vi "Bullet Markdown.vi"(8 "error in":errorcluster, 11 "File Path":path) -> (0 "error out":errorcluster, 2 "Wiki entry":string, 3 "Rendered metadata":string)   [LabVIEW 2020]
panel:
  out "result string":string
  out "String":string
  out "first subarray":string[](array[string])
  out "group/channel names":string[][](array[string])
  out "property values":variant[](array[variant])
  out "property names":string[](array[string])
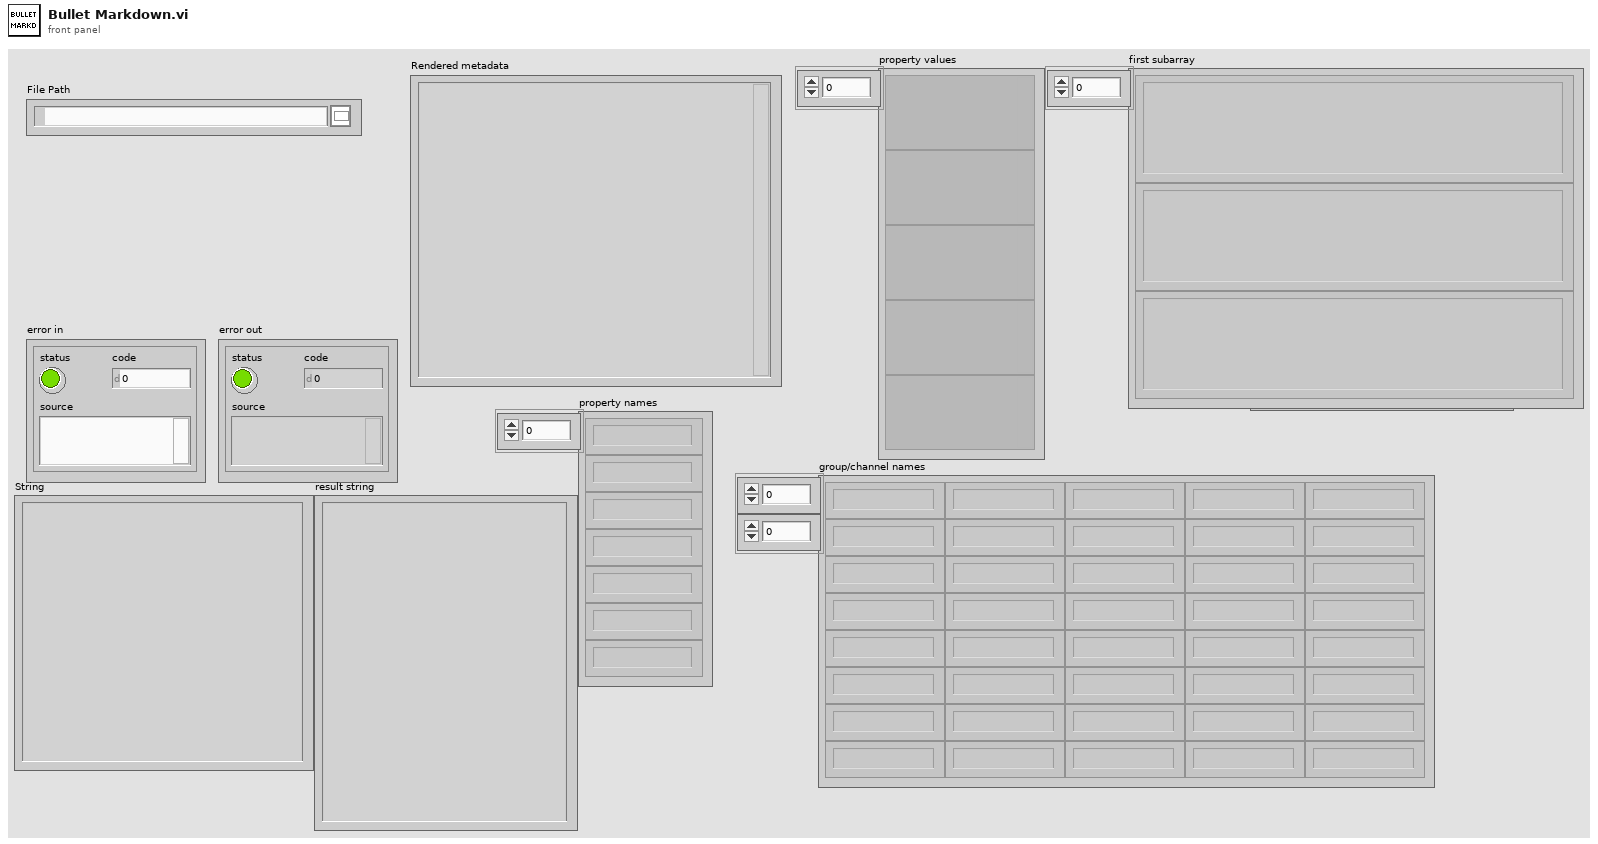
[diagram p1: front panel]
types:
  T1 = enum16{"open", "open or create", "create or replace", "create", "open (read-only)"}
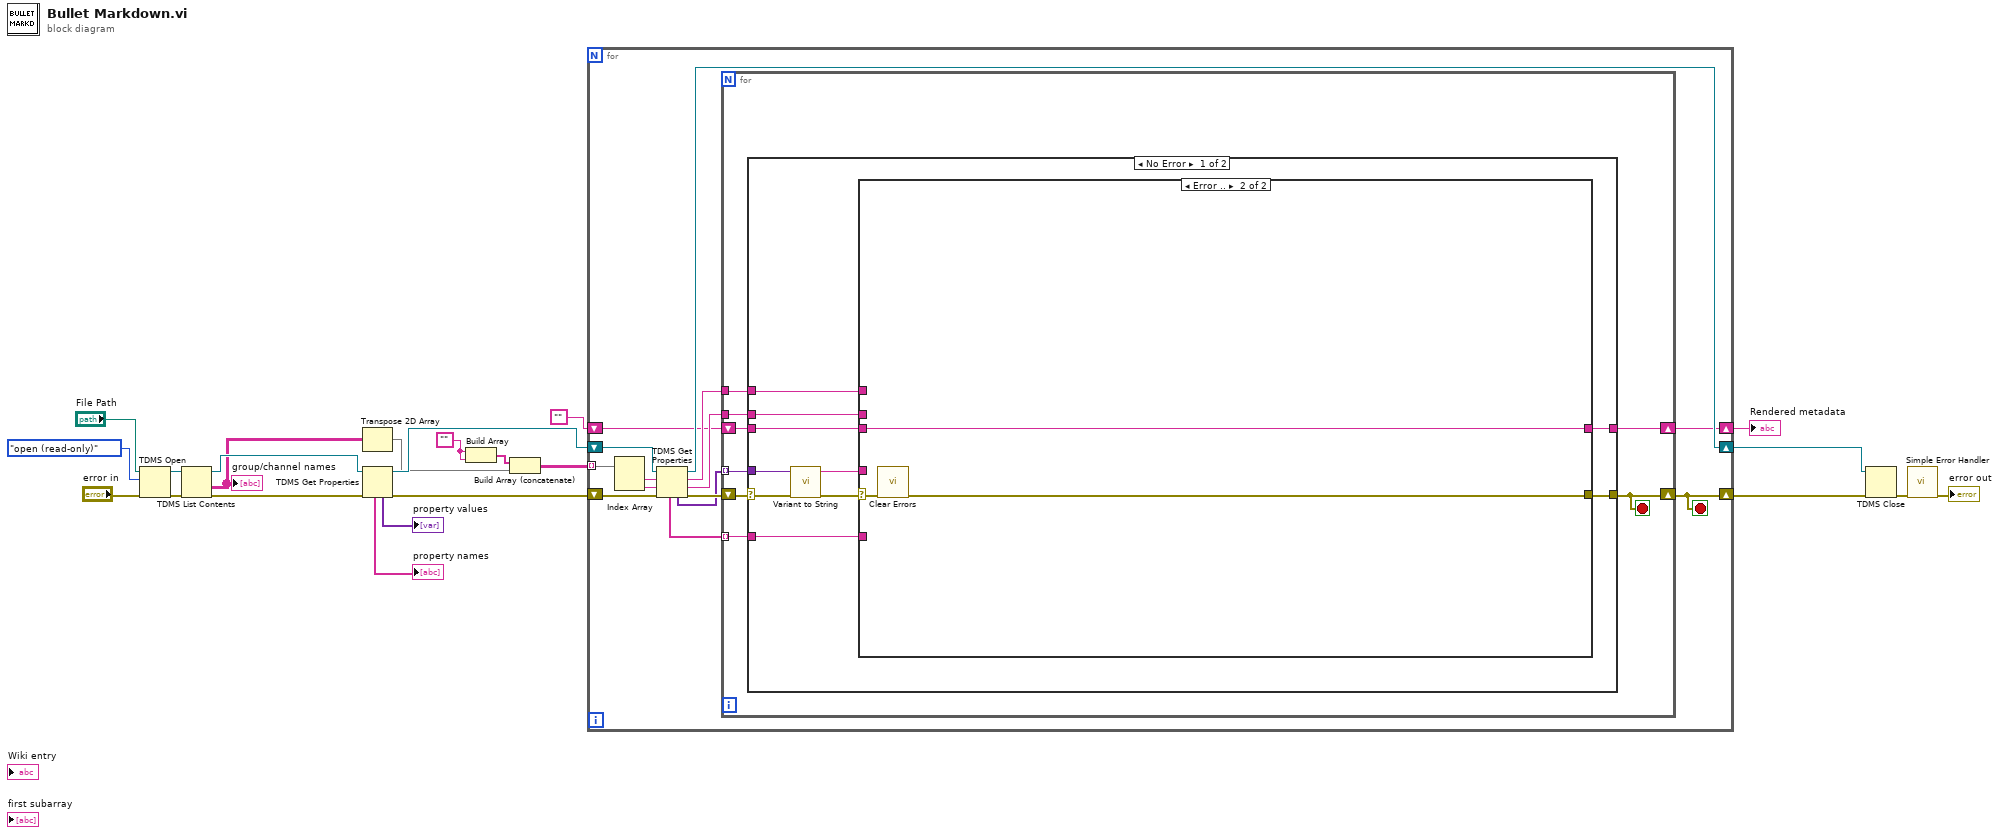
[diagram p0: block diagram]
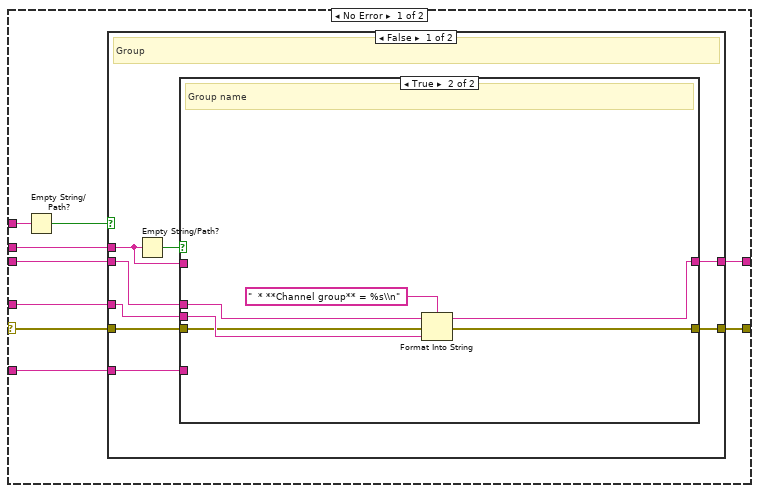
[diagram p2: hidden frame]
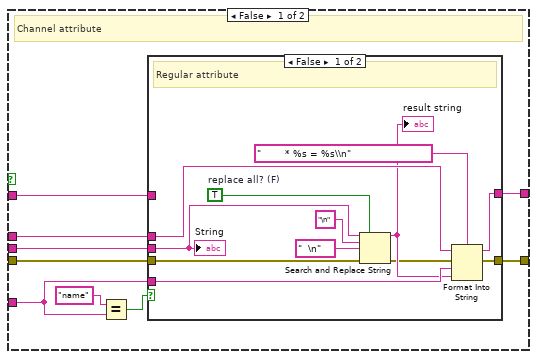
[diagram p3: hidden frame]
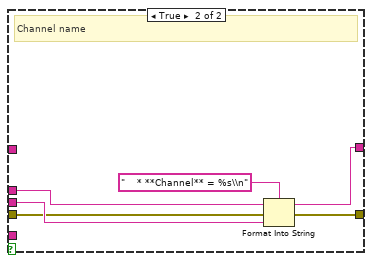
[diagram p4: hidden frame]
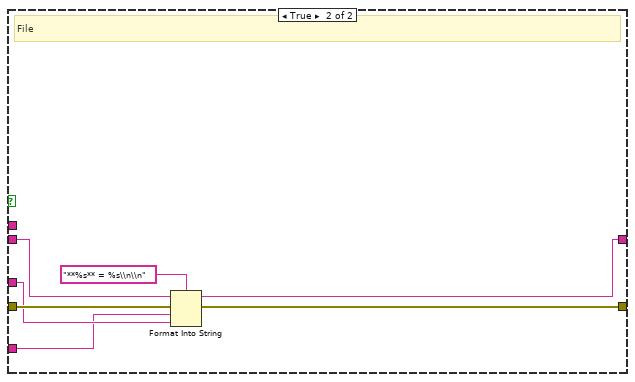
[diagram p5: hidden frame]
diagram:
  w5 = ""
  n1 = TDMS Open(8:"error in", 10:T1."open (read-only)" ("operation (0:open)"), 11:"File Path") -> (0:w16:errorcluster, 3:w14:refnum<k34>)  [unwired: 4 in]
  n2 = TDMS List Contents(4:w16, 7:w14) -> (0:w15:errorcluster, 1:w3:string[][], 3:w13:refnum<k34>)  [unwired: 1 in, 1 out]
  "group/channel names" <- w3
  n3 = Transpose 2D Array(2D array=w3) -> (transposed array=w2:string[][])
  n4 = TDMS Get Properties(8:w15, 11:w13) -> (0:w11:errorcluster, 3:w12:refnum<k34>, 4:→"property values":variant[], 6:→"property names":string[])  [unwired: 4 in, 2 out]
  n5 = Build Array(w5, w5) -> (w4:string[])
  n6 = Build Array (concatenate)(w4, w2) -> (w1:string[][])
  n7 = for {
    tunnel: w1 -> [w36] mode=indexing
    shift-right: [w31] -> w10
    shift-left: w12 -> [w33]
    shift-right: [w23] -> w9
    shift-left: w11 -> [w32]
    shift-right: [w25] -> w7
    shift-left: "" -> [w26]
    stop <- w23 stop-if-true
    n8 = Index Array(array=w36) -> (element #1=w35:string, element #2=w34:string)  [unwired: 2 in]
    n9 = TDMS Get Properties(8:w32, 9:w34, 10:w35, 11:w33) -> (0:w28:errorcluster, 1:w29:string, 2:w30:string, 3:w31:refnum<k34>, 4:w24:variant[], 6:w27:string[])  [unwired: 2 in]
    n10 = for {
      tunnel: w30 -> [w44]
      tunnel: w29 -> [w43]
      tunnel: w27 -> [w42] mode=indexing
      shift-right: [w38] -> w23
      shift-left: w28 -> [w39]
      shift-right: [w37] -> w25
      shift-left: w26 -> [w41]
      tunnel: w24 -> [w40] mode=indexing
      stop <- w38 stop-if-true
      n11 = case shown="No Error" w39 {
        selector: w39 -> [w45 w116]
        tunnel: w44 -> [w54 _]
        tunnel: w43 -> [w53 _]
        tunnel: [w52 w116] -> w38
        tunnel: w42 -> [w51 _]
        tunnel: w41 -> [w50 w115]
        tunnel: [w49 w115] -> w37
        tunnel: w40 -> [w46 _]
        frame No Error {
          n12 = call "Variant to String.vi"("error in"=w45, "Variant"=w46) -> ("error out"=w48:errorcluster, "Output string"=w47:string)  [unwired: 7 in, 1 out]
          n13 = case shown="Error .." w48 {
            selector: w48 -> [w55 w113]
            tunnel: w54 -> [w63 _]
            tunnel: w53 -> [w58 _]
            tunnel: [w56 w112] -> w52
            tunnel: w51 -> [w57 _]
            tunnel: w50 -> [w61 w114]
            tunnel: [w59 w114] -> w49
            tunnel: w47 -> [w60 _]
            frame No Error {
              n14 = Empty String/Path?(string/path=w63) -> (empty?=w62:bool)
              n15 = case shown="False" w62 {
                tunnel: w61 -> [w70 w111]
                tunnel: w60 -> [w69 w106]
                tunnel: [w68 w109] -> w59
                tunnel: w58 -> [w67 _]
                tunnel: w57 -> [w66 w105]
                tunnel: [w65 w108] -> w56
                tunnel: w55 -> [w64 w107]
                frame False {
                  # "Group"
                  n16 = Empty String/Path?(string/path=w67) -> (empty?=w71:bool)
                  n17 = case shown="True" w71 {
                    tunnel: w70 -> [w80 w103]
                    tunnel: w69 -> [w78 w102]
                    tunnel: [w77 w101] -> w68
                    tunnel: w67 -> [w79 _]
                    tunnel: w66 -> [w76 _]
                    tunnel: [w73 w100] -> w65
                    tunnel: w64 -> [w72 w99]
                    frame False {
                      # "Channel attribute"
                      n18 = Equal?(x="name", y=w76) -> (x = y?=w74:bool)
                      n19 = case shown="False" w74 {
                        tunnel: w80 -> [w91 w97]
                        tunnel: w79 -> [_ _]
                        tunnel: w76 -> [w90 _]
                        tunnel: w78 -> [w88 w95]
                        tunnel: [w89 w96] -> w77
                        tunnel: [w82 w94] -> w73
                        tunnel: w72 -> [w81 w93]
                        frame False {
                          w84 = TRUE  # replace all? (F)
                          # "Regular attribute"
                          n20 = Search and Replace String(replace all?=w84, input string=w88, search string="\n", replace string="  \n" ("replace string (\"\")"), error in=w81) -> (result string=w87:string, error out=w83:errorcluster)  [unwired: 3 in, 2 out]
                          "result string" <- w87
                          n21 = Format Into String(format string="        * %s = %s\\n", initial string=w91, error in=w83, w90, w87) -> (resulting string=w89:string, error out=w82:errorcluster)
                          "String" <- w88
                        }
                        frame True {
                          # "Channel name"
                          n22 = Format Into String(format string="    * **Channel** = %s\\n", initial string=w97, error in=w93, w95) -> (resulting string=w96:string, error out=w94:errorcluster)
                        }
                      }
                    }
                    frame True {
                      # "Group name"
                      n23 = Format Into String(format string="  * **Channel group** = %s\\n", initial string=w103, error in=w99, w102) -> (resulting string=w101:string, error out=w100:errorcluster)
                    }
                  }
                }
                frame True {
                  # "File"
                  n24 = Format Into String(format string="**%s** = %s\\n\\n", initial string=w111, error in=w107, w105, w106) -> (resulting string=w109:string, error out=w108:errorcluster)
                }
              }
            }
            frame Error {
              n25 = call <vilib>:"Clear Errors.vi"("error in (no error)"=w113) -> ("error out"=w112:errorcluster)  [unwired: 5 in, 1 out]
            }
          }
        }
        frame Error {
        }
      }
    }
  }
  "Rendered metadata" <- w7
  n26 = TDMS Close(8:w9, 11:w10) -> (0:w19:errorcluster)  [unwired: 1 out]
  n27 = call <vilib>:"Simple Error Handler.vi"("error in (no error)"=w19) -> ("error out"=→"error out":errorcluster)  [unwired: 4 in, 4 out]
